vi "read37(test_pro).vi"(0 "VISA资源名称":refnum<visa-resource-name>, 5 "Interval_ms":dbl=500.0, 7 "连接":bool) -> (2 "SENSOR23":dbl, 3 "SENSOR11":dbl, 4 "SENSOR1":dbl, 6 "SENSOR3":dbl, 8 "SENSOR5":dbl, 10 "SENSOR15":dbl, 13 "SENSOR21":dbl, 14 "SENSOR25":dbl, 15 "SENSOR13":dbl)   [LabVIEW 2017]
uses:
  <vilib>/Instr/_visa.llb/VISA Configure Serial Port (Instr).vi
  <vilib>/addons/Tools/Unicode/UTF8 Tools.lvlib
panel:
  out "错误输出":errorcluster
  out "错误输出 2":errorcluster caption="错误输出"
  in  "?":enum32{"CONTROL", "选项卡 2"}(tab)
  in  "停止按钮":bool
  in  "增益选择":u16(ring) items=["±6.144V", "±4.096V", "±2.048V", "±1.024V", "±0.512V", "±0.256V"]
  in  "连接方式":u16(ring) items=["Serial", "WiFi", "Dual"]
  out "数值显示控件 37":dbl
  out "数值显示控件":dbl
  out "数值显示控件 2":dbl
  out "数值显示控件 3":dbl
  out "数值显示控件 5":dbl
  out "数值显示控件 6":dbl
  out "数值显示控件 8":dbl
  out "数值显示控件 9":dbl
  out "数值显示控件 10":dbl
  out "数值显示控件 12":dbl
  out "数值显示控件 13":dbl
  out "数值显示控件 14":dbl
  out "数值显示控件 17":dbl
  out "数值显示控件 18":dbl
  out "数值显示控件 20":dbl
  out "数值显示控件 21":dbl
  out "数值显示控件 22":dbl
  out "数值显示控件 24":dbl
  out "数值显示控件 26":dbl
  out "数值显示控件 27":dbl
  out "数值显示控件 28":dbl
  out "数值显示控件 29":dbl
  out "数值显示控件 30":dbl
  out "数值显示控件 32":dbl
  out "数值显示控件 33":dbl
  out "数值显示控件 34":dbl
  out "数值显示控件 35":dbl
  out "数值显示控件 36":dbl
  out "本次":string
  out "finally":string[][](array[string])
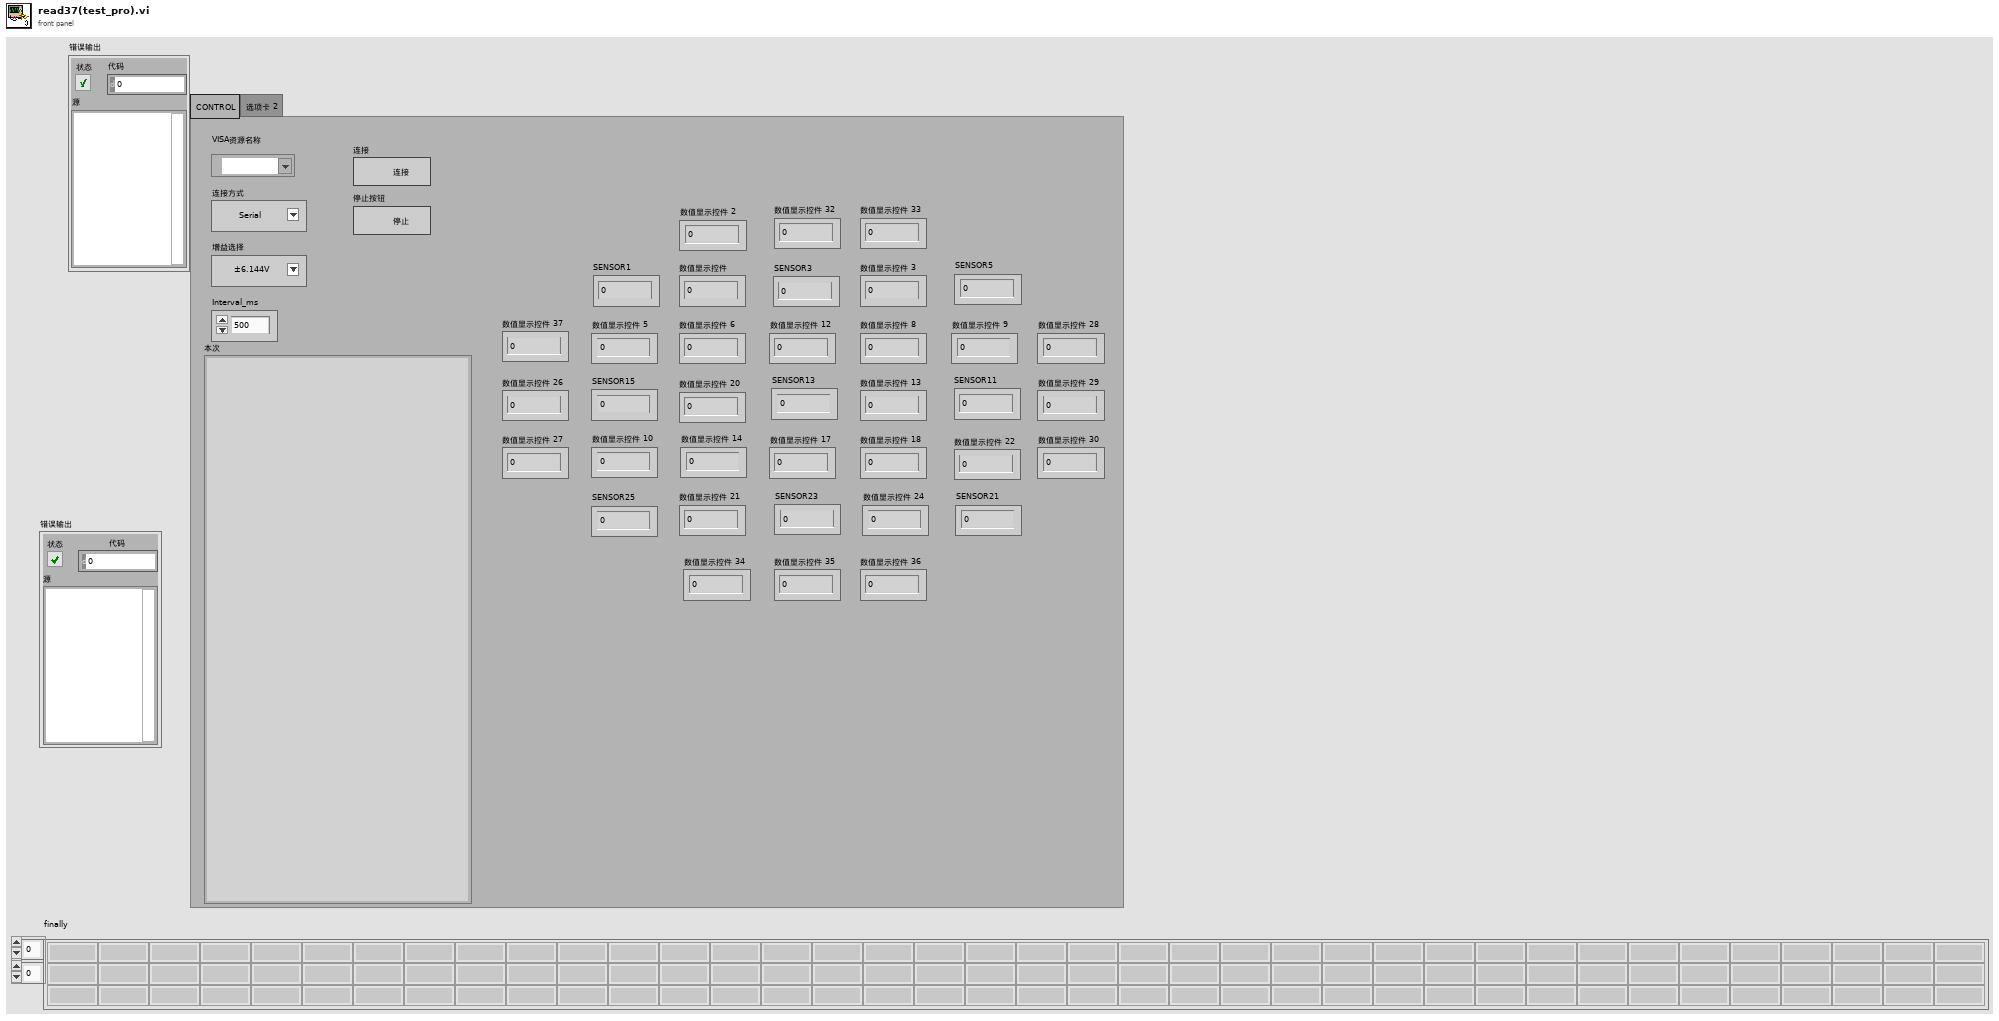
[diagram p1: front panel]
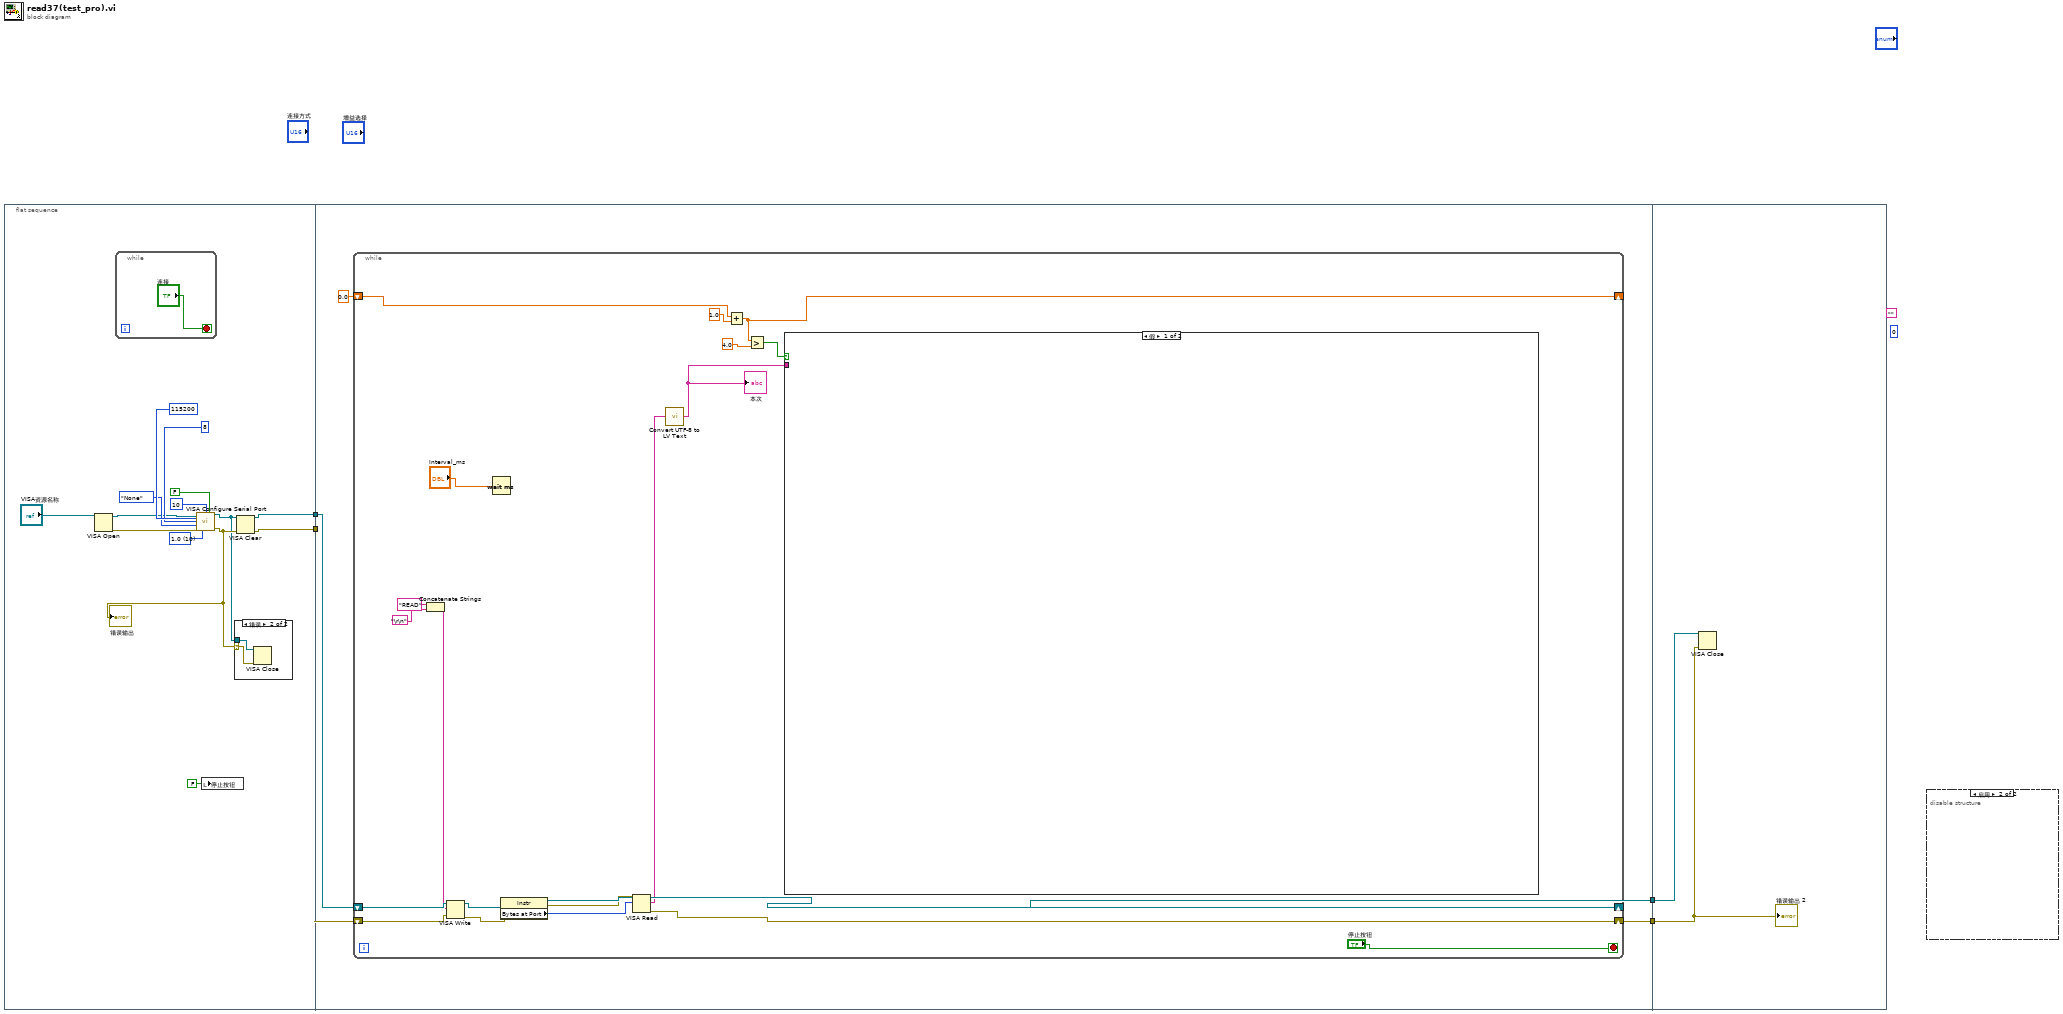
[diagram p0: block diagram]
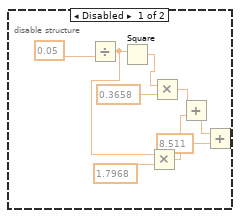
[diagram p2: hidden frame]
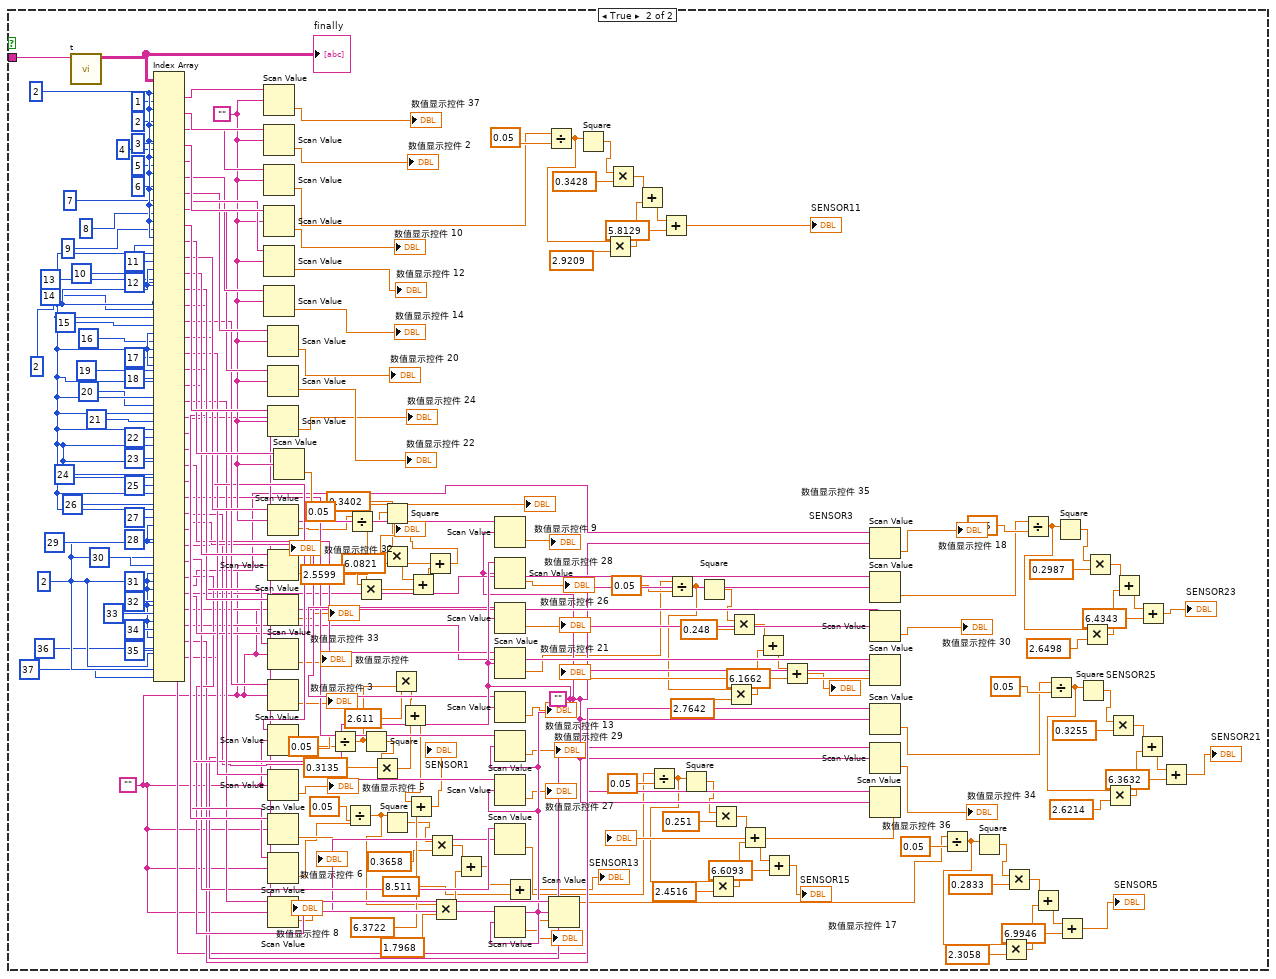
[diagram p4: hidden frame]
diagram:
  (unwired) 0
  (unwired) ""
  n1 = flat-sequence {
    tunnel: [w10] -> w4
    tunnel: [w11] -> w3
    tunnel: w4 -> [w26]
    tunnel: w3 -> [w25]
    tunnel: [w24] -> w2
    tunnel: [w23] -> w1
    tunnel: w2 -> [w258]
    tunnel: w1 -> [w257]
    frame #0 {
      w17 = u16 10 items=["1.0"=10, "1.5"=15, "2.0"=20] ("stop bits (10: 1 bit)")
      n2 = VISA Open(VISA resource name="VISA资源名称") -> (VISA resource name=w8:refnum<visa-resource-name>, error out=w7:errorcluster)  [unwired: 4 in]
      n3 = while {
        stop <- "连接" stop-if-true
      }
      n4 = call-poly "VISA Configure Serial Port"("VISA resource name"=w8, "termination char\n(0xA = '\\n' = LF)"=u8 10 ("termination char\n(0xA = '\\n' = LF)"), "Enable Termination\nChar (T)"=FALSE ("Enable Termination\nChar (T)"), "baud rate (9600)"=u32 115200, "data bits (8)"=u16 8, "parity (0:none)"=enum16{"None", "Odd", "Even", "Mark", "Space"}."None", "error in (no error)"=w7, "stop bits (10: 1 bit)"=w17) -> ("VISA resource name out"=w5:refnum<visa-resource-name>, "error out"=w6:errorcluster)  [unwired: 6 in]
      "错误输出" <- w6
      n5 = local write "停止按钮"(FALSE ("停止按钮")) -> ()
      n6 = case shown="错误" w6 {
        selector: w6 -> [_ w19]
        tunnel: w5 -> [_ w20]
        frame No Error {
        }
        frame Error {
          n7 = VISA Close(VISA resource name=w20, error in (no error)=w19) -> ()  [unwired: 1 out]
        }
      }
      n8 = VISA Clear(VISA resource name=w5, error in (no error)=w6) -> (VISA resource name out=w11:refnum<visa-resource-name>, error out=w10:errorcluster)
    }
    frame #1 {
      n9 = while {
        shift-right: [w44] -> w23
        shift-left: w26 -> [w47]
        shift-right: [w45] -> w24
        shift-left: w25 -> [w46]
        shift-right: [w34] -> _
        shift-left: 0.0 -> [w35]
        stop <- "停止按钮" stop-if-true
        n10 = Concatenate Strings("READ" ("字符串"), "\r\n") -> (w43:string)
        n11 = VISA Write(VISA resource name=w46, write buffer=w43, error in (no error)=w47) -> (VISA resource name out=w42:refnum<visa-resource-name>, error out=w41:errorcluster)  [unwired: 1 out]
        n12 = Wait (ms)(milliseconds to wait="Interval_ms") -> ()  [unwired: 1 out]
        n13 = property class="Instr"(reference=w42, error in=w41) -> (reference out=w39:refnum<visa-resource-name>, error out=w38:errorcluster, "Bytes at Port"=w37:u32)
        n14 = VISA Read(VISA resource name=w39, byte count=w37, error in (no error)=w38) -> (VISA resource name out=w45:refnum<visa-resource-name>, read buffer=w36:string, error out=w44:errorcluster)  [unwired: 1 out]
        n15 = call <vilib>:"Convert UTF-8 to LV Text.vi"("UTF-8 Text"=w36) -> ("LV Text"=w27:string)  [unwired: 13 in, 1 out]
        "本次" <- w27
        n16 = Add(x=w35, y=1.0) -> (x+y=w34:dbl)
        n17 = Greater?(x=w34, y=4.0) -> (0:w30:bool)
        n18 = case shown="假" w30 {
          tunnel: w27 -> [_ w48]
          frame False {
          }
          frame True {
            w167 = ""
            w168 = ""
            w199 = 2 ("索引 (行)")
            w225 = 2 ("索引 (行)")
            w195 = ""
            w255 = 2 ("索引 (行)")
            n19 = call "t.vi"("待处理字符串"=w48) -> ("finally"=w256:string[][])  [unwired: 10 in]
            "finally" <- w256
            n20 = Index Array(array=w256, index (row) #1=w255, index (col) #1=1 ("禁用的索引 (列)"), index (row) #2=w255, index (col) #2=2 ("禁用的索引 (列)"), index (row) #3=w255, index (col) #3=3 ("禁用的索引 (列)"), index (row) #4=w255, index (col) #4=4 ("禁用的索引 (列)"), index (row) #5=w255, index (col) #5=5 ("禁用的索引 (列)"), index (row) #6=w255, index (col) #6=6 ("禁用的索引 (列)"), index (row) #7=w255, index (col) #7=7 ("禁用的索引 (列)"), index (row) #8=w255, index (col) #8=8 ("禁用的索引 (列)"), index (row) #9=w255, index (col) #9=9 ("禁用的索引 (列)"), index (row) #10=w255, index (col) #10=10 ("禁用的索引 (列)"), index (row) #11=w225, index (col) #11=11 ("禁用的索引 (列)"), index (row) #12=w225, index (col) #12=12 ("禁用的索引 (列)"), index (row) #13=w225, index (col) #13=13 ("禁用的索引 (列)"), index (row) #14=w225, index (col) #14=14 ("禁用的索引 (列)"), index (row) #15=w225, index (col) #15=15 ("禁用的索引 (列)"), index (row) #16=w225, index (col) #16=16 ("禁用的索引 (列)"), index (row) #17=w225, index (col) #17=17 ("禁用的索引 (列)"), index (row) #18=w225, index (col) #18=18 ("禁用的索引 (列)"), index (row) #19=w225, index (col) #19=19 ("禁用的索引 (列)"), index (row) #20=w225, index (col) #20=20 ("禁用的索引 (列)"), index (row) #21=w225, index (col) #21=21 ("禁用的索引 (列)"), index (row) #22=w225, index (col) #22=22 ("禁用的索引 (列)"), index (row) #23=w225, index (col) #23=23 ("禁用的索引 (列)"), index (row) #24=w225, index (col) #24=24 ("禁用的索引 (列)"), index (row) #25=w225, index (col) #25=25 ("禁用的索引 (列)"), index (row) #26=w225, index (col) #26=26 ("禁用的索引 (列)"), index (row) #27=w225, index (col) #27=27 ("禁用的索引 (列)"), index (row) #28=w199, index (col) #28=28 ("禁用的索引 (列)"), index (row) #29=w199, index (col) #29=29 ("禁用的索引 (列)"), index (row) #30=w199, index (col) #30=30 ("禁用的索引 (列)"), index (row) #31=w199, index (col) #31=31 ("禁用的索引 (列)"), index (row) #32=w199, index (col) #32=32 ("禁用的索引 (列)"), index (row) #33=w199, index (col) #33=33 ("禁用的索引 (列)"), index (row) #34=w199, index (col) #34=34 ("禁用的索引 (列)"), index (row) #35=w199, index (col) #35=35 ("禁用的索引 (列)"), index (row) #36=w199, index (col) #36=36 ("禁用的索引 (列)"), index (row) #37=w199, index (col) #37=37 ("禁用的索引 (列)")) -> (element #1=w247:string, element #2=w246:string, element #3=w245:string, element #4=w244:string, element #5=w243:string, element #6=w242:string, element #7=w241:string, element #8=w240:string, element #9=w236:string, element #10=w235:string, element #11=w196:string, element #12=w194:string, element #13=w193:string, element #14=w192:string, element #15=w191:string, element #16=w190:string, element #17=w189:string, element #18=w188:string, element #19=w187:string, element #20=w186:string, element #21=w185:string, element #22=w184:string, element #23=w183:string, element #24=w182:string, element #25=w181:string, element #26=w180:string, element #27=w179:string, element #28=w178:string, element #29=w177:string, element #30=w176:string, element #31=w175:string, element #32=w174:string, element #33=w173:string, element #34=w172:string, element #35=w171:string, element #36=w170:string, element #37=w169:string)
            n21 = Scan Value(string=w247, format string=w195) -> (value=→"数值显示控件 37":dbl)  [unwired: 1 in, 1 out]
            n22 = Scan Value(string=w246, format string=w195) -> (value=→"数值显示控件 2":dbl)  [unwired: 1 in, 1 out]
            n23 = Scan Value(string=w245, format string=w195) -> (value=w85:dbl)  [unwired: 1 in, 1 out]
            n24 = Scan Value(string=w244, format string=w195) -> (value=→"数值显示控件 10":dbl)  [unwired: 1 in, 1 out]
            n25 = Scan Value(string=w243, format string=w195) -> (value=→"数值显示控件 12":dbl)  [unwired: 1 in, 1 out]
            n26 = Scan Value(string=w242, format string=w195) -> (value=→"数值显示控件 14":dbl)  [unwired: 1 in, 1 out]
            n27 = Scan Value(string=w241, format string=w195) -> (value=→"数值显示控件 20":dbl)  [unwired: 1 in, 1 out]
            n28 = Scan Value(string=w240, format string=w195) -> (value=→"数值显示控件 22":dbl)  [unwired: 1 in, 1 out]
            n29 = Scan Value(string=w236, format string=w195) -> (value=→"数值显示控件 24":dbl)  [unwired: 1 in, 1 out]
            n30 = Scan Value(string=w196, format string=w195) -> (value=w136:dbl)  [unwired: 1 in, 1 out]
            n31 = Scan Value(string=w194, format string=w168) -> (value=→"数值显示控件 32":dbl)  [unwired: 1 in, 1 out]
            n32 = Scan Value(string=w193, format string=w168) -> (value=→"数值显示控件 33":dbl)  [unwired: 1 in, 1 out]
            n33 = Scan Value(string=w192, format string=w168) -> (value=→"数值显示控件":dbl)  [unwired: 1 in, 1 out]
            n34 = Scan Value(string=w191, format string=w168) -> (value=→"数值显示控件 3":dbl)  [unwired: 1 in, 1 out]
            n35 = Scan Value(string=w190, format string=w168) -> (value=w147:dbl)  [unwired: 1 in, 1 out]
            n36 = Scan Value(string=w189, format string=w168) -> (value=→"数值显示控件 5":dbl)  [unwired: 1 in, 1 out]
            n37 = Scan Value(string=w188, format string=w168) -> (value=→"数值显示控件 6":dbl)  [unwired: 1 in, 1 out]
            n38 = Scan Value(string=w187, format string=w168) -> (value=w95:dbl)  [unwired: 1 in, 1 out]
            n39 = Scan Value(string=w186, format string=w168) -> (value=→"数值显示控件 8":dbl)  [unwired: 1 in, 1 out]
            n40 = Scan Value(string=w235, format string=w195) -> (value=→"数值显示控件 35":dbl)  [unwired: 1 in, 1 out]
            n41 = Divide(x=w147, y=0.05) -> (x/y=w142:dbl)
            n42 = Divide(x=w95, y=0.05) -> (x/y=w102:dbl)
            n43 = Divide(x=w136, y=0.05) -> (x/y=w131:dbl)
            n44 = Multiply(x=w131, y=2.5599) -> (x*y=w129:dbl)
            n45 = Square(x=w142) -> (x^2=w145:dbl)
            n46 = Multiply(x=w145, y=0.3135) -> (x*y=w143:dbl)
            n47 = Square(x=w131) -> (x^2=w134:dbl)
            n48 = Multiply(x=w134, y=0.3402) -> (x*y=w132:dbl)
            n49 = Square(x=w102) -> (x^2=w100:dbl)
            n50 = Multiply(x=2.611, y=w142) -> (x*y=w140:dbl)
            n51 = Add(x=w140, y=w143) -> (x+y=w139:dbl)
            n52 = Add(x=w139, y=6.3722) -> (x+y=→"SENSOR1":dbl)
            n53 = Add(x=w132, y=w129) -> (x+y=w128:dbl)
            n54 = Add(x=6.0821, y=w128) -> (x+y=→"SENSOR3":dbl)
            n55 = Multiply(x=w100, y=0.3658) -> (x*y=w101:dbl)
            n56 = Multiply(x=w102, y=1.7968) -> (x*y=w103:dbl)
            n57 = Add(x=w101, y=w103) -> (x+y=w50:dbl)
            n58 = Scan Value(string=w185, format string=w167) -> (value=→"数值显示控件 9":dbl)  [unwired: 1 in, 1 out]
            n59 = Scan Value(string=w184, format string=w167) -> (value=→"数值显示控件 28":dbl)  [unwired: 1 in, 1 out]
            n60 = Scan Value(string=w183, format string=w167) -> (value=→"数值显示控件 26":dbl)  [unwired: 1 in, 1 out]
            n61 = Scan Value(string=w182, format string=w167) -> (value=w74:dbl)  [unwired: 1 in, 1 out]
            n62 = Scan Value(string=w181, format string=w167) -> (value=→"数值显示控件 13":dbl)  [unwired: 1 in, 1 out]
            n63 = Scan Value(string=w180, format string=w167) -> (value=→"数值显示控件 29":dbl)  [unwired: 1 in, 1 out]
            n64 = Scan Value(string=w179, format string=w167) -> (value=→"数值显示控件 27":dbl)  [unwired: 1 in, 1 out]
            n65 = Scan Value(string=w178, format string=w167) -> (value=w105:dbl)  [unwired: 1 in, 1 out]
            n66 = Scan Value(string=w176, format string=w167) -> (value=→"数值显示控件 17":dbl)  [unwired: 1 in, 1 out]
            n67 = Add(x=w50, y=8.511) -> (x+y=→"SENSOR13":dbl)
            n68 = Divide(x=w85, y=0.05) -> (x/y=w90:dbl)
            n69 = Scan Value(string=w177, format string=w167) -> (value=w116:dbl)  [unwired: 1 in, 1 out]
            n70 = Square(x=w90) -> (x^2=w93:dbl)
            n71 = Multiply(x=w90, y=2.9209) -> (x*y=w88:dbl)
            n72 = Multiply(x=w93, y=0.3428) -> (x*y=w91:dbl)
            n73 = Add(x=w91, y=w88) -> (x+y=w87:dbl)
            n74 = Divide(x=w105, y=0.05) -> (x/y=w110:dbl)
            n75 = Add(x=w87, y=5.8129) -> (x+y=→"SENSOR11":dbl)
            n76 = Divide(x=w74, y=0.05) -> (x/y=w80:dbl)
            n77 = Square(x=w110) -> (x^2=w113:dbl)
            n78 = Square(x=w80) -> (x^2=w83:dbl)
            n79 = Multiply(x=w110, y=2.4516) -> (x*y=w108:dbl)
            n80 = Multiply(x=w113, y=0.251) -> (x*y=w111:dbl)
            n81 = Multiply(x=w80, y=2.7642) -> (x*y=w78:dbl)
            n82 = Multiply(x=w83, y=0.248) -> (x*y=w81:dbl)
            n83 = Add(x=w111, y=w108) -> (x+y=w107:dbl)
            n84 = Add(x=w81, y=w78) -> (x+y=w77:dbl)
            n85 = Add(x=w107, y=6.6093) -> (x+y=→"SENSOR15":dbl)
            n86 = Add(x=w77, y=6.1662) -> (x+y=→"SENSOR25":dbl)
            n87 = Scan Value(string=w175, format string=w167) -> (value=→"数值显示控件 18":dbl)  [unwired: 1 in, 1 out]
            n88 = Scan Value(string=w174, format string=w167) -> (value=w63:dbl)  [unwired: 1 in, 1 out]
            n89 = Scan Value(string=w173, format string=w167) -> (value=→"数值显示控件 30":dbl)  [unwired: 1 in, 1 out]
            n90 = Scan Value(string=w172, format string=w167) -> (value=→"数值显示控件 21":dbl)  [unwired: 1 in, 1 out]
            n91 = Scan Value(string=w171, format string=w167) -> (value=w52:dbl)  [unwired: 1 in, 1 out]
            n92 = Scan Value(string=w170, format string=w167) -> (value=→"数值显示控件 34":dbl)  [unwired: 1 in, 1 out]
            n93 = Scan Value(string=w169, format string=w167) -> (value=→"数值显示控件 36":dbl)  [unwired: 1 in, 1 out]
            n94 = Divide(x=w116, y=0.05) -> (x/y=w121:dbl)
            n95 = Square(x=w121) -> (x^2=w124:dbl)
            n96 = Multiply(x=w121, y=2.3058) -> (x*y=w119:dbl)
            n97 = Multiply(x=w124, y=0.2833) -> (x*y=w122:dbl)
            n98 = Divide(x=w63, y=0.05) -> (x/y=w70:dbl)
            n99 = Add(x=w122, y=w119) -> (x+y=w118:dbl)
            n100 = Divide(x=w52, y=0.05) -> (x/y=w59:dbl)
            n101 = Square(x=w70) -> (x^2=w68:dbl)
            n102 = Add(x=w118, y=6.9946) -> (x+y=→"SENSOR5":dbl)
            n103 = Square(x=w59) -> (x^2=w57:dbl)
            n104 = Multiply(x=w70, y=2.6498) -> (x*y=w71:dbl)
            n105 = Multiply(x=w68, y=0.2987) -> (x*y=w69:dbl)
            n106 = Multiply(x=w59, y=2.6214) -> (x*y=w60:dbl)
            n107 = Multiply(x=w57, y=0.3255) -> (x*y=w58:dbl)
            n108 = Add(x=w69, y=w71) -> (x+y=w72:dbl)
            n109 = Add(x=w58, y=w60) -> (x+y=w61:dbl)
            n110 = Add(x=w72, y=6.4343) -> (x+y=→"SENSOR23":dbl)
            n111 = Add(x=w61, y=6.3632) -> (x+y=→"SENSOR21":dbl)
          }
        }
      }
    }
    frame #2 {
      n112 = VISA Close(VISA resource name=w258, error in (no error)=w257) -> ()  [unwired: 1 out]
      "错误输出 2" <- w257
    }
  }
  n113 = disable-structure shown="启用" {
    frame Disabled {
      n114 = Divide(y=0.05) -> (x/y=w263:dbl)  [unwired: 1 in]
      n115 = Square(x=w263) -> (x^2=w266:dbl)
      n116 = Multiply(x=w263, y=1.7968) -> (x*y=w261:dbl)
      n117 = Multiply(x=w266, y=0.3658) -> (x*y=w264:dbl)
      n118 = Add(x=w264, y=w261) -> (x+y=w260:dbl)
      n119 = Add(x=w260, y=8.511) -> ()  [unwired: 1 out]
    }
    frame Enabled {
    }
  }
